vi "PTSequencer.panel.vi"() -> ()   [LabVIEW 2014, in "PTSequencer.lvlib"]
uses:
  PTSequencer.lvlib
  PTSequencer.mode.ctl
  CSlibraries/UtilityLib/UtilityLib.helpType.ctl
  CS_Core/CSSystem/CoreLib/CoreLib.string 2 byte array.vi
  CSlibraries/UtilityLib/UtilityLib.lvlib
  _common/PTUtils/PTUtils.lvlib
  CS_Core/BaseSM/BaseSM.lvlib
  CS_Core/BaseProcess/BaseProcess.lvlib
  CS_Core/CSSystem/CSSystemLib/CSSystemLib.lvlib
  CS_Core/CSSystem/CoreLib/CoreLib.lvlib
  CS_Core/CSObj/CSObj.lvlib
panel:
  out "Paused":bool
  in  "settings path":path caption="Settings file"
  out "objlist_OldVal":i32[](array[numeric])
  in  "nofLoops":u32 caption="##"
  out "Current loop":i32 caption="Loop"
  out "running":bool
  out "Current step":i32 caption="Step"
  out "State":string
  in  "Mode":T1 caption="Mode:"
  out "Busy":bool
  out "error out":errorcluster
  in  "error in (no error)":errorcluster
  in  "object ref":refnum<vi>
  out "loop counter":i32
  in  "Tab":enum32{"Sequence", "Log"}(tab)
  in  "object list":i32[](listbox)
  out "Status Log":string
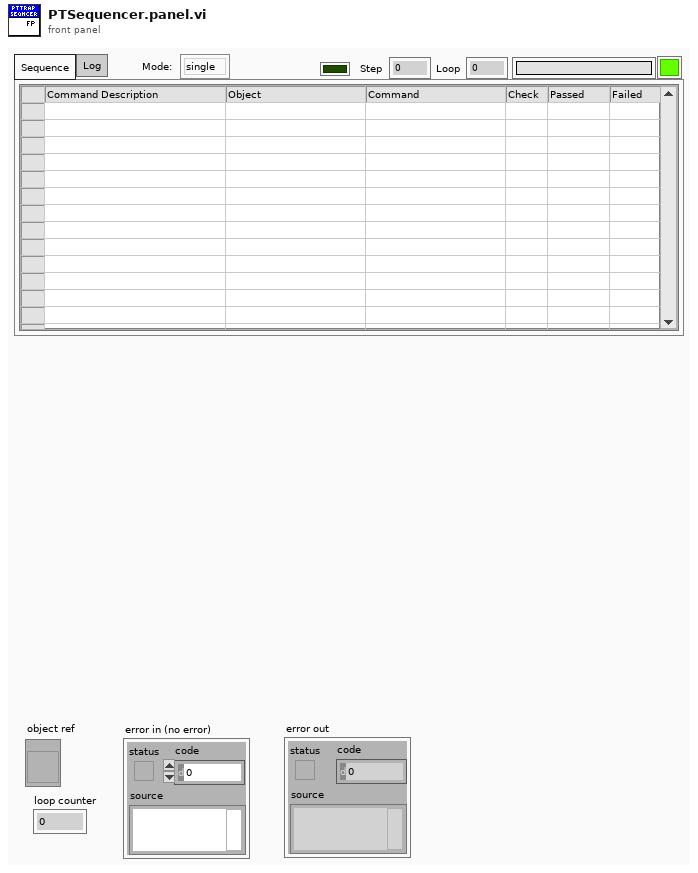
[diagram p1: front panel]
types:
  T1 = typedef "PTSequencer.lvlib/PTSequencer.mode.ctl" = enum16{"single", "loop", "for loop"}
  T2 = enum16{"open", "replace", "create", "open or create", "replace or create", "replace or create with confirmation"}
  T3 = typedef "UtilityLib.lvlib/UtilityLib.helpType.ctl" = enum16{"unknown", "menu", "description", "about", "special0", "special1", "special2"}
  T4 = typedef "PTSequencer.lvlib/PTSequencer.i attribute.ctl" = cluster{"subsequence":bool, "mode":T1, "i step":i32, "nofLoops":i32, "i loop":i32, "Running":bool, "Paused":bool, "step done":bool, "loop done":bool, "seq done":bool, "DIM IDs":cluster{"step done":i32, "loop done":i32, "seq done":i32, "i step":i32, "i loop":i32}, "use stop conditions":bool, "stop conditions":T5[], "Step List":T7[], "DIM subsriptions":string[], "stop cond indexes":i32[], "step cond indexes":cluster{"step condition IDs":cluster{"step ID":i32, "condition ID":i32}[]}[], "Delay Start Time":timestamp, "status":string, "stopping":bool}
  T5 = typedef "PTSequencer.lvlib/PTSequencer.DIM service condition.ctl" = cluster{"DIM service":string, "descr":string, "nomValue":T6, "actValue":T6, "matched":bool, "DIM Status":cluster{"no link":bool, "quality":i32, "Time Stamp":timestamp}}
  T6 = typedef "CoreDefs.rawDataType.ctl" = i8[]
  T7 = typedef "PTSequencer.lvlib/PTSequencer.step.ctl" = cluster{"description":string, "object parameters":cluster{"object":string, "selector":string, "descriptor":string, "data":T6, "subsequence":bool, "call mode":enum16{"Simple DIM", "Synchronous"}, "data in":T6}, "result action":cluster{"check":bool, "passed":enum16{"Next", "Previous", "Repeat", "Jump"}, "failed":enum16{"Next", "Previous", "Repeat", "Jump"}, "jumpID_passed":i32, "jumpID_failed":i32}, "conditions":T5[], "fulfilled ":bool, "use delay":bool, "delay time (s)":dbl, "ID":i32}
  T8 = typedef "eventvkey.ctl" = enum16{"ASCII", "Enter", "Return", "Shift", "Ctrl", "Alt", "Cmd", "Opt", "Caps", "NumLock", "Clear", "Break", "Up", "Down", "Left", "Right", "Insert", "Delete", "Home", "End", "PageUp", "PageDown", "Escape", "Help", "Pause", "ScrollLock", "F1", "F2", "F3", "F4", "F5", "F6", "F7", "F8", "F9", "F10", "F11", "F12", "F13", "F14", "F15", "F16", "F17", "F18", "F19", "F20", "F21", "F22", "F23", "F24", "Play", "VolumeUp", "VolumeDown", "Mute", "Two Byte Char"}
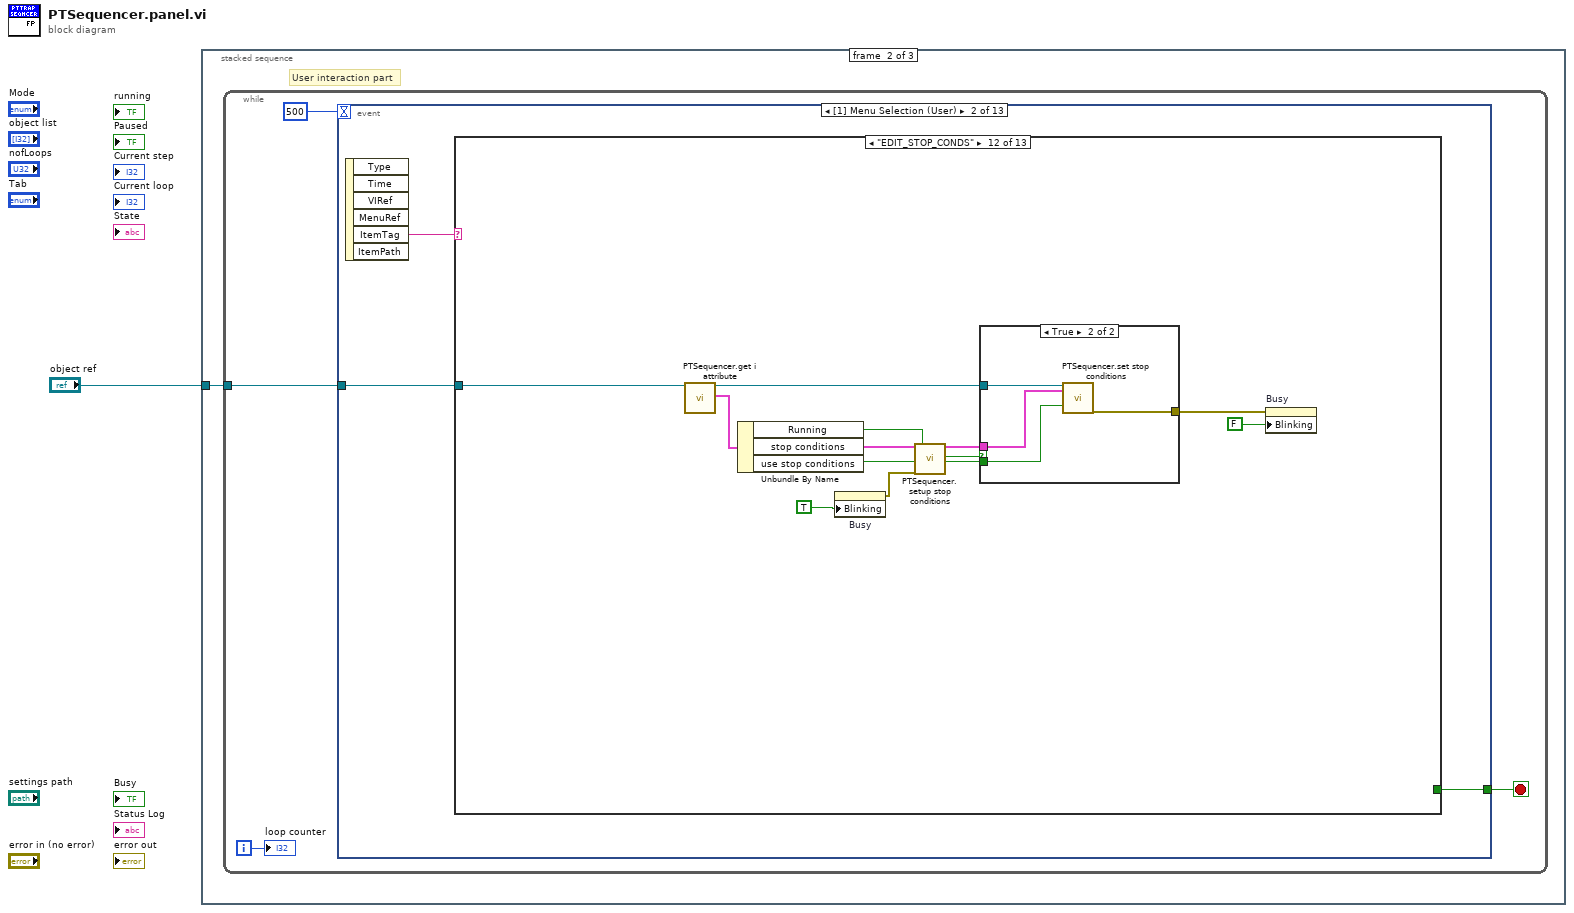
[diagram p0: block diagram]
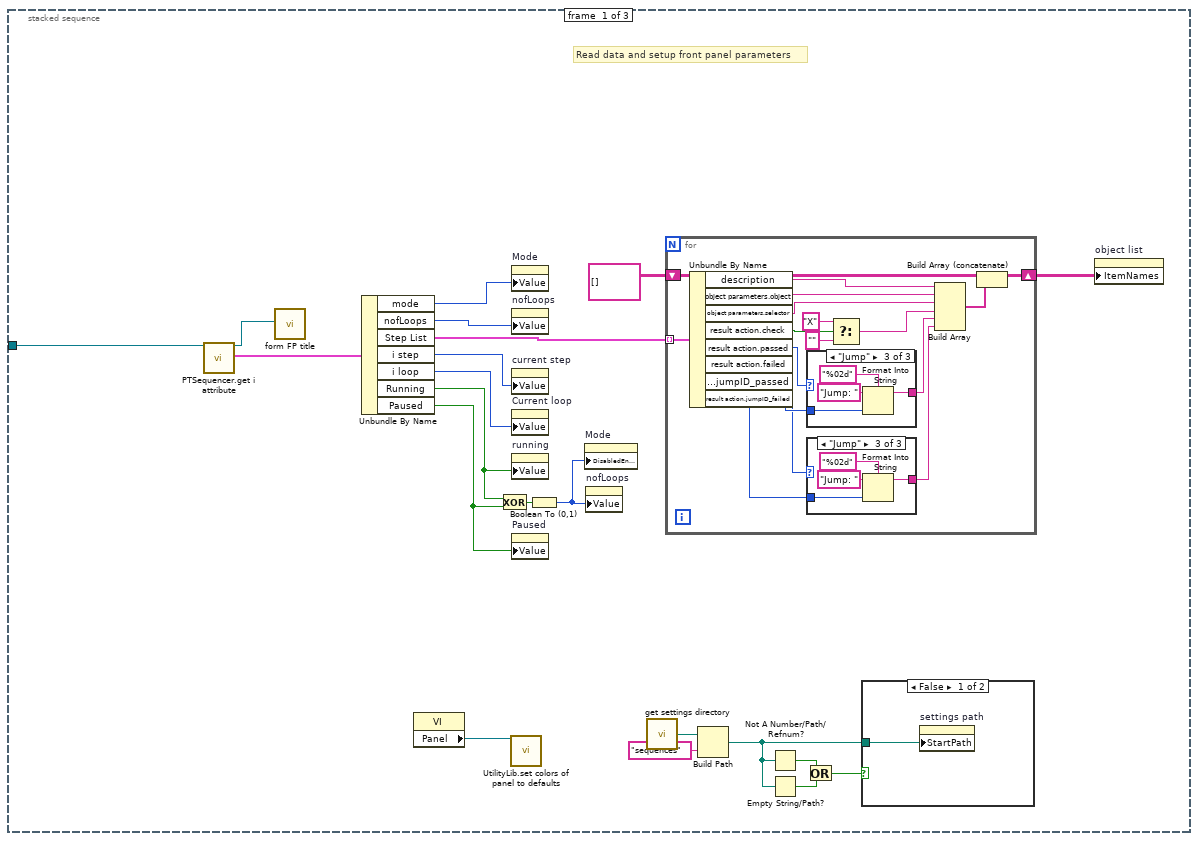
[diagram p2: hidden frame]
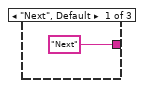
[diagram p3: hidden frame]
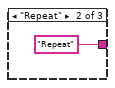
[diagram p4: hidden frame]
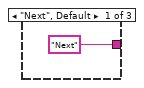
[diagram p5: hidden frame]
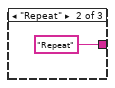
[diagram p6: hidden frame]
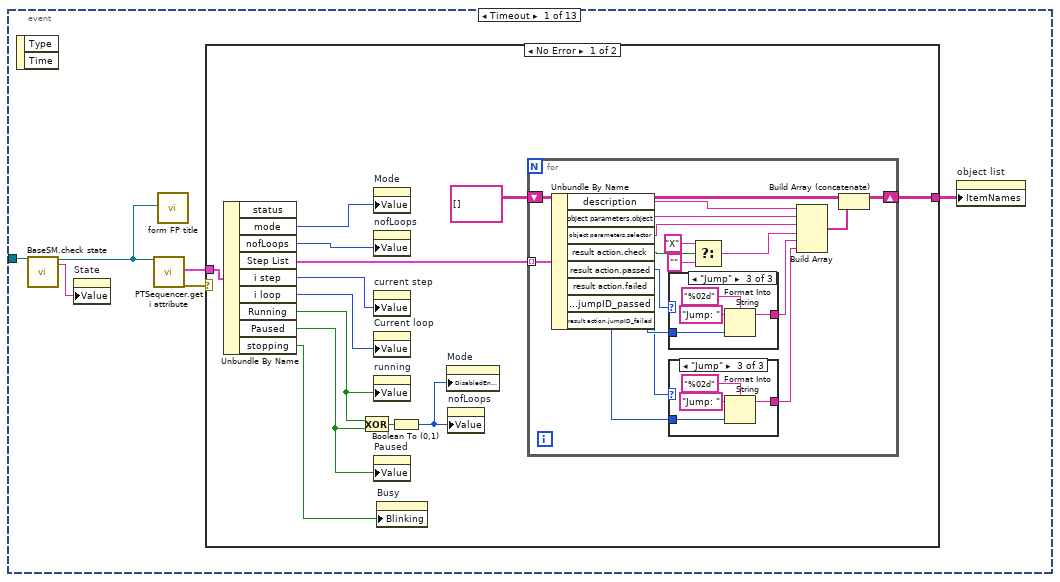
[diagram p8: hidden frame]
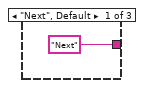
[diagram p9: hidden frame]
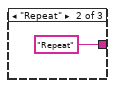
[diagram p10: hidden frame]
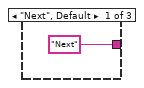
[diagram p11: hidden frame]
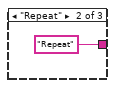
[diagram p12: hidden frame]
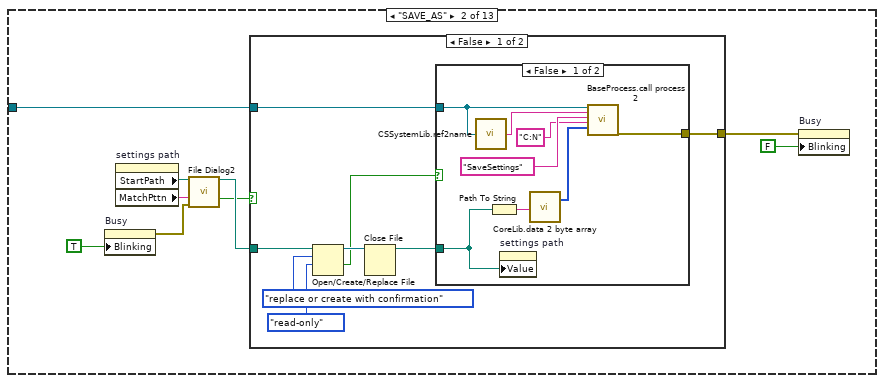
[diagram p15: hidden frame]
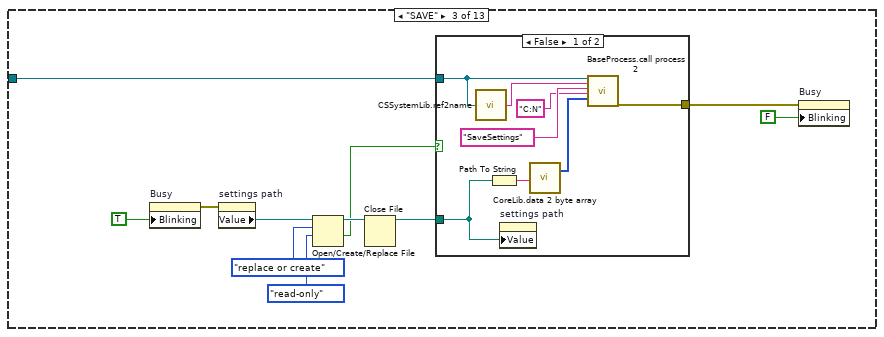
[diagram p18: hidden frame]
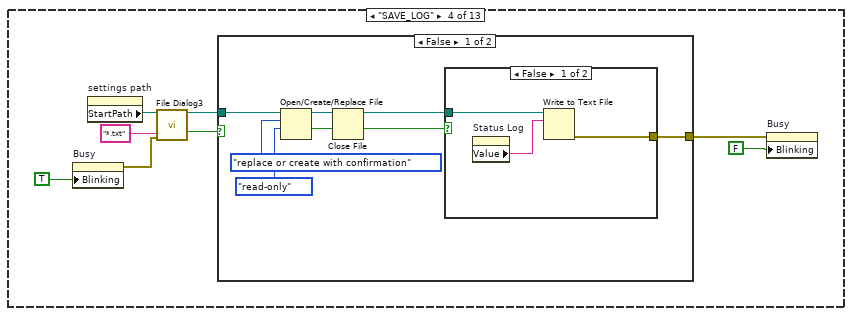
[diagram p20: hidden frame]
diagram:
  n1 = stacked-sequence {
    tunnel: "object ref" -> [w13 w53 w388]
    frame #0 {
      # "Read data and setup front panel parameters"
      n2 = call "PTSequencer.get i attribute.vi"("i ref in"=w13) -> ("i ref out"=w2:refnum<vi>, "i attribute"=w14:T4)  [unwired: 16 in, 1 out]
      n3 = call "form FP title.vi"("object ref"=w2) -> ()  [unwired: 19 in]
      n4 = Unbundle By Name(w14) -> ("mode"=w6:T1, "nofLoops"=w5:i32, "Step List"=w10:T7[], "i step"=w11:i32, "i loop"=w9:i32, "Running"=w4:bool, "Paused"=w7:bool)
      n5 = property class="VI"() -> ("Panel"=w16:refnum<vi>)  [unwired: 2 in, 2 out]
      n6 = Exclusive Or(1:w7, 2:w4) -> (0:w8:bool)
      n7 = call "UtilityLib.set colors of panel to defaults.vi"("Front Panel"=w16) -> ()  [unwired: 18 in, 1 out]
      n8 = property on="Mode" class="Enum (strict)"("Value"=w6) -> ()  [unwired: 2 in, 2 out]
      n9 = property on="nofLoops" class="DigNum (strict)"("Value"=w5) -> ()  [unwired: 2 in, 2 out]
      n10 = property on="current step" class="DigNum (strict)"("Value"=w11) -> ()  [unwired: 2 in, 2 out]
      n11 = property on="Current loop" class="DigNum (strict)"("Value"=w9) -> ()  [unwired: 2 in, 2 out]
      n12 = property on="running" class="Bool (strict)"("Value"=w4) -> ()  [unwired: 2 in, 2 out]
      n13 = property on="Paused" class="Bool (strict)"("Value"=w7) -> ()  [unwired: 2 in, 2 out]
      n14 = Boolean To (0,1)(Boolean=w8) -> (0, 1=w3:i16)
      n15 = property on="Mode" class="Enum (strict)"("DisabledEnum"=w3) -> ()  [unwired: 2 in, 2 out]
      n16 = property on="nofLoops" class="DigNum (strict)"("Value"=w3) -> ()  [unwired: 2 in, 2 out]
      n17 = call "get settings directory.vi"() -> ("settings directory"=w19:path)
      n18 = for {
        shift-right: [w38] -> w15
        shift-left: string[][] [] -> [w39]
        tunnel: w10 -> [w37] mode=indexing
        n19 = Unbundle By Name(w37) -> ("description"=w36:string, "object parameters.object"=w34:string, "object parameters.selector"=w33:string, "result action.check"=w32:bool, "result action.passed"=w27:enum16{"Next", "Previous", "Repeat", "Jump"}, "result action.failed"=w24:enum16{"Next", "Previous", "Repeat", "Jump"}, "result action.jumpID_passed"=w26:i32, "result action.jumpID_failed"=w23:i32)
        n20 = case shown="\"Jump\"" w27 {
          tunnel: ["Next" "Repeat" w50] -> w28
          tunnel: w26 -> [_ _ w49]
          frame "Next", Default {
          }
          frame "Repeat" {
          }
          frame "Jump" {
            n21 = Format Into String(format string="%02d", initial string="Jump: ", w49) -> (resulting string=w50:string)  [unwired: 1 in, 1 out]
          }
        }
        n22 = case shown="\"Jump\"" w24 {
          tunnel: ["Next" "Repeat" w44] -> w25
          tunnel: w23 -> [_ _ w43]
          frame "Next", Default {
          }
          frame "Repeat" {
          }
          frame "Jump" {
            n23 = Format Into String(format string="%02d", initial string="Jump: ", w43) -> (resulting string=w44:string)  [unwired: 1 in, 1 out]
          }
        }
        n24 = Select(t="X", s=w32, f="") -> (s? t:f=w29:string)
        n25 = Build Array(w36, w34, w33, w29, w28, w25) -> (w35:string[])
        n26 = Build Array (concatenate)(w39, w35) -> (w38:string[][])
      }
      n27 = Build Path(base path=w19, name or relative path="sequences") -> (appended path=w17:path)
      n28 = Not A Number/Path/Refnum?(number/path/refnum=w17) -> (NaN/Path/Refnum?=w22:bool)
      n29 = Empty String/Path?(string/path=w17) -> (empty?=w21:bool)
      n30 = Or(x=w22, y=w21) -> (x .or. y?=w20:bool)
      n31 = case shown="False" w20 {
        tunnel: w17 -> [w52 _]
        frame False {
          n32 = property on="settings path" class="Path"("StartPath"=w52) -> ()  [unwired: 2 in, 2 out]
        }
        frame True {
        }
      }
      n33 = property on="object list" class="MCListbox (strict)"("ItemNames"=w15) -> ()  [unwired: 2 in, 2 out]
    }
    frame #1 {
      # "User interaction part"
      n34 = while {
        tunnel: w53 -> [w54]
        i -> [w57]
        stop <- w55 stop-if-true
        n35 = event shown="[1] Menu Selection (User)" {
          selector: _ -> [_ _ _ _ _ _ _ _ _ _ _ _ _]
          dyn-events: _ -> [_ _ _ _ _ _ _ _ _ _ _ _ _]
          timeout: 500 -> [_ _ _ _ _ _ _ _ _ _ _ _ _]
          tunnel: [_ w106 _ _ _ _ _ _ _ _ _ _ _] -> w55
          tunnel: w54 -> [w63 w107 w238 _ w268 w318 w335 _ w354 w360 w369 w379 w385]
          event Timeout {
            n36 = event-data() -> ()  [unwired: 1 in, 2 out]
            n37 = call "BaseSM.check state.vi"("i ref in"=w63) -> ("i ref out"=w59:refnum<vi>, "actualState"=w60:string)  [unwired: 13 in, 4 out]
            n38 = property on="State" class="Str"("Value"=w60) -> ()  [unwired: 2 in, 2 out]
            n39 = call "PTSequencer.get i attribute.vi"("i ref in"=w59) -> ("i attribute"=w61:T4, "error out"=w58:errorcluster)  [unwired: 16 in, 1 out]
            n40 = call "form FP title.vi"("object ref"=w59) -> ()  [unwired: 19 in]
            n41 = case shown="No Error" w58 {
              tunnel: [w76 _] -> w62
              tunnel: w61 -> [w75 _]
              frame No Error {
                n42 = Unbundle By Name(w75) -> ("mode"=w68:T1, "nofLoops"=w67:i32, "Step List"=w72:T7[], "i step"=w73:i32, "i loop"=w71:i32, "Running"=w66:bool, "Paused"=w69:bool, "stopping"=w64:bool)  [unwired: 1 out]
                n43 = Exclusive Or(1:w69, 2:w66) -> (0:w70:bool)
                n44 = property on="Mode" class="Enum (strict)"("Value"=w68) -> ()  [unwired: 2 in, 2 out]
                n45 = property on="nofLoops" class="DigNum (strict)"("Value"=w67) -> ()  [unwired: 2 in, 2 out]
                n46 = property on="current step" class="DigNum (strict)"("Value"=w73) -> ()  [unwired: 2 in, 2 out]
                n47 = property on="Current loop" class="DigNum (strict)"("Value"=w71) -> ()  [unwired: 2 in, 2 out]
                n48 = property on="running" class="Bool (strict)"("Value"=w66) -> ()  [unwired: 2 in, 2 out]
                n49 = property on="Paused" class="Bool (strict)"("Value"=w69) -> ()  [unwired: 2 in, 2 out]
                n50 = property on="Busy" class="Bool (strict)"("Blinking"=w64) -> ()  [unwired: 2 in, 2 out]
                n51 = Boolean To (0,1)(Boolean=w70) -> (0, 1=w65:i16)
                n52 = property on="Mode" class="Enum (strict)"("DisabledEnum"=w65) -> ()  [unwired: 2 in, 2 out]
                n53 = property on="nofLoops" class="DigNum (strict)"("Value"=w65) -> ()  [unwired: 2 in, 2 out]
                n54 = for {
                  shift-right: [w92] -> w76
                  shift-left: string[][] [] -> [w93]
                  tunnel: w72 -> [w91] mode=indexing
                  n55 = Unbundle By Name(w91) -> ("description"=w90:string, "object parameters.object"=w88:string, "object parameters.selector"=w87:string, "result action.check"=w86:bool, "result action.passed"=w81:enum16{"Next", "Previous", "Repeat", "Jump"}, "result action.failed"=w78:enum16{"Next", "Previous", "Repeat", "Jump"}, "result action.jumpID_passed"=w80:i32, "result action.jumpID_failed"=w77:i32)
                  n56 = case shown="\"Jump\"" w81 {
                    tunnel: ["Next" "Repeat" w104] -> w82
                    tunnel: w80 -> [_ _ w103]
                    frame "Next", Default {
                    }
                    frame "Repeat" {
                    }
                    frame "Jump" {
                      n57 = Format Into String(format string="%02d", initial string="Jump: ", w103) -> (resulting string=w104:string)  [unwired: 1 in, 1 out]
                    }
                  }
                  n58 = case shown="\"Jump\"" w78 {
                    tunnel: ["Next" "Repeat" w98] -> w79
                    tunnel: w77 -> [_ _ w97]
                    frame "Next", Default {
                    }
                    frame "Repeat" {
                    }
                    frame "Jump" {
                      n59 = Format Into String(format string="%02d", initial string="Jump: ", w97) -> (resulting string=w98:string)  [unwired: 1 in, 1 out]
                    }
                  }
                  n60 = Select(t="X", s=w86, f="") -> (s? t:f=w83:string)
                  n61 = Build Array(w90, w88, w87, w83, w82, w79) -> (w89:string[])
                  n62 = Build Array (concatenate)(w93, w89) -> (w92:string[][])
                }
              }
              frame Error {
              }
            }
            n63 = property on="object list" class="MCListbox (strict)"("ItemNames"=w62) -> ()  [unwired: 2 in, 2 out]
          }
          event Menu Selection (User) {
            n64 = event-data() -> ("ItemTag"=w108:string)  [unwired: 1 in, 5 out]
            n65 = case shown="\"EDIT_STOP_CONDS\"" w108 {
              tunnel: w107 -> [_ w113 w144 _ w182 _ w193 w195 w198 w201 w206 w223 _]
              tunnel: [_ _ _ _ _ TRUE _ _ _ _ _ _ _] -> w106
              frame "", Default {
              }
              frame "SAVE_AS" {
                n66 = property on="Busy" class="Bool (strict)"("Blinking"=TRUE) -> (error out=w109:errorcluster)  [unwired: 2 in, 1 out]
                n67 = property on="settings path" class="Path"() -> ("StartPath"=w117:path, "MatchPttn"=w116:string)  [unwired: 2 in, 2 out]
                n68 = call "File Dialog2"("start path"=w117, "error in"=w109, "pattern (all files)"=w116) -> ("selected path"=w115:path, "cancelled"=w114:bool)  [unwired: 9 in, 2 out]
                n69 = case shown="False" w114 {
                  tunnel: w115 -> [w124 _]
                  tunnel: w113 -> [w125 _]
                  tunnel: [w118 _] -> w111
                  frame False {
                    n70 = Open/Create/Replace File(file path (use dialog)=w124, operation (0:open)=T2."replace or create with confirmation", access (0:read/write)=enum16{"read/write", "read-only", "write-only"}."read-only") -> (refnum out=w123:refnum<file>, cancelled=w121:bool)  [unwired: 3 in, 1 out]
                    n71 = Close File(refnum=w123) -> (path=w122:path)  [unwired: 1 in, 1 out]
                    n72 = case shown="False" w121 {
                      tunnel: w122 -> [w127 _]
                      tunnel: w125 -> [w129 _]
                      tunnel: [w126 _] -> w118
                      frame False {
                        n73 = call "CSSystemLib.ref2name.vi"("obj refnum"=w129) -> ("name"=w128:string)
                        n74 = Path To String(path=w127) -> (string=w130:string)
                        n75 = property on="settings path" class="Path"("Value"=w127) -> ()  [unwired: 2 in, 2 out]
                        n76 = call-poly "CoreLib.data 2 byte array.vi"("string"=w130) -> ("byteArray out"=w131:T6)  [unwired: 18 in]
                        n77 = call "BaseProcess.call process 2.vi"("i ref in"=w129, "Object"=w128, "Selector"="SaveSettings", "Data Descriptor"="C:N", "Data"=w131) -> ("error out"=w126:errorcluster)  [unwired: 13 in, 1 out]
                      }
                      frame True {
                      }
                    }
                  }
                  frame True {
                  }
                }
                n78 = property on="Busy" class="Bool (strict)"(error in=w111, "Blinking"=FALSE) -> ()  [unwired: 1 in, 2 out]
              }
              frame "SAVE" {
                n79 = property on="Busy" class="Bool (strict)"("Blinking"=TRUE) -> (error out=w139:errorcluster)  [unwired: 2 in, 1 out]
                n80 = property on="settings path" class="Path"(error in=w139) -> ("Value"=w140:path)  [unwired: 1 in, 2 out]
                n81 = Open/Create/Replace File(file path (use dialog)=w140, operation (0:open)=T2."replace or create", access (0:read/write)=enum16{"read/write", "read-only", "write-only"}."read-only") -> (refnum out=w138:refnum<file>, cancelled=w136:bool)  [unwired: 3 in, 1 out]
                n82 = Close File(refnum=w138) -> (path=w137:path)  [unwired: 1 in, 1 out]
                n83 = case shown="False" w136 {
                  tunnel: w137 -> [w146 _]
                  tunnel: w144 -> [w148 _]
                  tunnel: [w145 _] -> w142
                  frame False {
                    n84 = call "CSSystemLib.ref2name.vi"("obj refnum"=w148) -> ("name"=w147:string)
                    n85 = Path To String(path=w146) -> (string=w149:string)
                    n86 = property on="settings path" class="Path"("Value"=w146) -> ()  [unwired: 2 in, 2 out]
                    n87 = call-poly "CoreLib.data 2 byte array.vi"("string"=w149) -> ("byteArray out"=w150:T6)  [unwired: 18 in]
                    n88 = call "BaseProcess.call process 2.vi"("i ref in"=w148, "Object"=w147, "Selector"="SaveSettings", "Data Descriptor"="C:N", "Data"=w150) -> ("error out"=w145:errorcluster)  [unwired: 13 in, 1 out]
                  }
                  frame True {
                  }
                }
                n89 = property on="Busy" class="Bool (strict)"(error in=w142, "Blinking"=FALSE) -> ()  [unwired: 1 in, 2 out]
              }
              frame "SAVE_LOG" {
                n90 = property on="Busy" class="Bool (strict)"("Blinking"=TRUE) -> (error out=w154:errorcluster)  [unwired: 2 in, 1 out]
                n91 = property on="settings path" class="Path"() -> ("StartPath"=w160:path)  [unwired: 2 in, 2 out]
                n92 = call "File Dialog3"("start path"=w160, "error in"=w154, "pattern (all files)"="*.txt" ("default name")) -> ("selected path"=w159:path, "cancelled"=w158:bool)  [unwired: 9 in, 2 out]
                n93 = case shown="False" w158 {
                  tunnel: w159 -> [w167 _]
                  tunnel: [w161 _] -> w156
                  frame False {
                    n94 = Open/Create/Replace File(file path (use dialog)=w167, operation (0:open)=T2."replace or create with confirmation", access (0:read/write)=enum16{"read/write", "read-only", "write-only"}."read-only") -> (refnum out=w166:refnum<file>, cancelled=w164:bool)  [unwired: 3 in, 1 out]
                    n95 = Close File(refnum=w166) -> (path=w165:path)  [unwired: 1 in, 1 out]
                    n96 = case shown="False" w164 {
                      tunnel: w165 -> [w168 _]
                      tunnel: [w169 _] -> w161
                      frame False {
                        n97 = property on="Status Log" class="Str"() -> ("Value"=w170:string)  [unwired: 2 in, 2 out]
                        n98 = Write to Text File(file (use dialog)=w168, text=w170) -> (error out=w169:errorcluster)  [unwired: 2 in, 2 out]
                      }
                      frame True {
                      }
                    }
                  }
                  frame True {
                  }
                }
                n99 = property on="Busy" class="Bool (strict)"(error in=w156, "Blinking"=FALSE) -> ()  [unwired: 1 in, 2 out]
              }
              frame "LOAD" {
                n100 = property on="settings path" class="Path"() -> ("StartPath"=w181:path, "MatchPttn"=w180:string)  [unwired: 2 in, 2 out]
                n101 = property on="Busy" class="Bool (strict)"("Blinking"=TRUE) -> (error out=w171:errorcluster)  [unwired: 2 in, 1 out]
                n102 = call "File Dialog"("start path"=w181, "error in"=w171, "pattern (all files)"=w180) -> ("selected path"=w179:path, "exists"=w175:bool, "cancelled"=w177:bool)  [unwired: 9 in, 1 out]
                n103 = Not(x=w175) -> (.not. x?=w178:bool)
                n104 = Or(x=w178, y=w177) -> (x .or. y?=w176:bool)
                n105 = case shown="False" w176 {
                  tunnel: w182 -> [w187 _]
                  tunnel: w179 -> [w185 _]
                  tunnel: [w183 _] -> w172
                  frame False {
                    n106 = call "CSSystemLib.ref2name.vi"("obj refnum"=w187) -> ("name"=w188:string)
                    n107 = Path To String(path=w185) -> (string=w186:string)
                    n108 = property on="settings path" class="Path"("Value"=w185) -> ()  [unwired: 2 in, 2 out]
                    n109 = call-poly "CoreLib.data 2 byte array.vi"("string"=w186) -> ("byteArray out"=w189:T6)  [unwired: 18 in]
                    n110 = call "BaseProcess.call process 1.vi"("i ref in"=w187, "Object"=w188, "Selector"="LoadSettings", "CallType"=enum16{"simple", "synchronous", "asynchronous"}."synchronous", "Data"=w189, "Data Descriptor"="C:N") -> ("error out"=w183:errorcluster)  [unwired: 11 in, 2 out]
                  }
                  frame True {
                  }
                }
                n111 = property on="Busy" class="Bool (strict)"(error in=w172, "Blinking"=FALSE) -> ()  [unwired: 1 in, 2 out]
              }
              frame "QUIT" {
              }
              frame "Hide" {
                n112 = call "CSObj.open front panel.vi"("i ref in"=w193, "frontPanelOpen"=FALSE ("front panel open")) -> ()  [unwired: 16 in, 2 out]
              }
              frame "START" {
                n113 = call "CSSystemLib.ref2name.vi"("obj refnum"=w195) -> ("name"=w197:string)
                n114 = call "BaseProcess.call process 2.vi"("i ref in"=w195, "Object"=w197, "Selector"="Start") -> ()  [unwired: 15 in, 2 out]
              }
              frame "STOP" {
                n115 = call "CSSystemLib.ref2name.vi"("obj refnum"=w198) -> ("name"=w200:string)
                n116 = call "BaseProcess.call process 2.vi"("i ref in"=w198, "Object"=w200, "Selector"="Stop") -> ()  [unwired: 15 in, 2 out]
              }
              frame "ABORT" {
                n117 = call "CSSystemLib.ref2name.vi"("obj refnum"=w201) -> ("name"=w203:string)
                n118 = call "BaseProcess.call process 2.vi"("i ref in"=w201, "Object"=w203, "Selector"="Abort") -> ()  [unwired: 15 in, 2 out]
              }
              frame "PAUSE" {
                n119 = property on="Paused" class="Bool (strict)"() -> ("Value"=w205:bool)  [unwired: 2 in, 2 out]
                n120 = Not(x=w205) -> (.not. x?=w204:bool)
                n121 = case shown="True" w204 {
                  tunnel: w206 -> [w209 w212]
                  frame True {
                    n122 = call "CSSystemLib.ref2name.vi"("obj refnum"=w209) -> ("name"=w208:string)
                    n123 = call "BaseProcess.call process 2.vi"("i ref in"=w209, "Object"=w208, "Selector"="Pause") -> ()  [unwired: 15 in, 2 out]
                  }
                  frame False {
                    n124 = call "CSSystemLib.ref2name.vi"("obj refnum"=w212) -> ("name"=w211:string)
                    n125 = call "BaseProcess.call process 2.vi"("i ref in"=w212, "Object"=w211, "Selector"="Start") -> ()  [unwired: 15 in, 2 out]
                  }
                }
              }
              frame "EDIT_STOP_CONDS" {
                n126 = call "PTSequencer.get i attribute.vi"("i ref in"=w223) -> ("i ref out"=w224:refnum<vi>, "i attribute"=w225:T4)  [unwired: 16 in, 1 out]
                n127 = Unbundle By Name(w225) -> ("Running"=w213:bool, "stop conditions"=w220:T5[], "use stop conditions"=w219:bool)
                n128 = property on="Busy" class="Bool (strict)"("Blinking"=TRUE) -> (error out=w214:errorcluster)  [unwired: 2 in, 1 out]
                n129 = call "PTSequencer.setup stop conditions.vi"("stop conditions in"=w220, "Use stop conditions in"=w219, "error in (no error)"=w214, "read only"=w213) -> ("stop conditions out"=w217:T5[], "changed"=w216:bool, "Use stop conditions out"=w218:bool)  [unwired: 12 in, 1 out]
                n130 = case shown="True" w216 {
                  tunnel: w218 -> [_ w228]
                  tunnel: w217 -> [_ w229]
                  tunnel: w224 -> [_ w227]
                  tunnel: [_ w226] -> w221
                  frame False {
                  }
                  frame True {
                    n131 = call "PTSequencer.set stop conditions.vi"("i ref in"=w227, "stop conditions"=w229, "use stop conditions"=w228) -> ("error out"=w226:errorcluster)  [unwired: 14 in, 2 out]
                  }
                }
                n132 = property on="Busy" class="Bool (strict)"(error in=w221, "Blinking"=FALSE) -> ()  [unwired: 1 in, 2 out]
              }
              frame "helpDescription" {
                n133 = call "UtilityLib.show help.vi"("helpType"=UtilityLib.helpType."description") -> ()
              }
            }
          }
          event Menu Activation? {
            n134 = event-data() -> ("MenuRef"=w244:refnum<k9>)  [unwired: 1 in, 3 out]
            n135 = call "PTSequencer.get i attribute.vi"("i ref in"=w238) -> ("i attribute"=w237:T4)  [unwired: 16 in, 2 out]
            n136 = Unbundle By Name(w237) -> ("Step List"=w236:T7[])
            n137 = Array Size(array=w236) -> (size(s)=w235:i32)
            n138 = Greater Than 0?(x=w235) -> (x > 0?=w234:bool)
            n139 = property on="running" class="Bool (strict)"() -> ("Value"=w253:bool)  [unwired: 2 in, 2 out]
            n140 = property on="settings path" class="Path"() -> ("Value"=w240:path)  [unwired: 2 in, 2 out]
            n141 = Empty String/Path?(string/path=w240) -> (empty?=w242:bool)
            n142 = Not A Number/Path/Refnum?(number/path/refnum=w240) -> (NaN/Path/Refnum?=w241:bool)
            n143 = Not(x=w253) -> (.not. x?=w239:bool)
            n144 = Not Or(1:w241, 2:w242) -> (0:w233:bool)
            n145 = And(x=w234, y=w239) -> (x .and. y?=w232:bool)
            n146 = And(x=w233, y=w232) -> (x .and. y?=w231:bool)
            n147 = Set Menu Item Info(7:"SAVE", 9:w231, 11:w244) -> (3:w243:refnum<k9>)  [unwired: 4 in, 1 out]
            n148 = Set Menu Item Info(7:"SAVE_AS", 9:w232, 11:w243) -> (3:w256:refnum<k9>)  [unwired: 4 in, 1 out]
            n149 = property on="Status Log" class="Str"() -> ("Value"=w250:string)  [unwired: 2 in, 2 out]
            n150 = Set Menu Item Info(7:"LOAD", 9:w239, 11:w256) -> (3:w252:refnum<k9>)  [unwired: 4 in, 1 out]
            n151 = call <vilib>:"Trim Whitespace.vi"("string"=w250) -> ("trimmed string"=w251:string)  [unwired: 1 in]
            n152 = property on="Paused" class="Bool (strict)"() -> ("Value"=w254:bool)  [unwired: 2 in, 2 out]
            n153 = Empty String/Path?(string/path=w251) -> (empty?=w247:bool)
            n154 = Set Menu Item Info(6:w254, 7:"PAUSE", 9:w253, 11:w252) -> (3:w248:refnum<k9>)  [unwired: 3 in, 1 out]
            n155 = Not(x=w247) -> (.not. x?=w246:bool)
            n156 = Set Menu Item Info(7:"SAVE_LOG", 9:w246, 11:w248) -> ()  [unwired: 4 in, 2 out]
            n157 = event-data() -> ()  [unwired: 2 in, 1 out]
          }
          event "object list": Shortcut Menu Activation? {
            n158 = event-data() -> ("MenuRef"=w259:refnum<k9>)  [unwired: 1 in]
            n159 = property on="object list" class="MCListbox (strict)"() -> ("Value"=w261:i32[])  [unwired: 2 in, 2 out]
            n160 = Array Size(array=w261) -> (size(s)=w260:i32)
            n161 = case shown="0, Default" w260 {
              tunnel: w259 -> [w263 w266]
              frame 0, Default {
                n162 = Set Menu Item Info(7:"CMD_EDIT", 9:FALSE, 11:w263) -> ()  [unwired: 4 in, 2 out]
              }
              frame 1 {
                n163 = Set Menu Item Info(7:"CMD_EDIT", 9:TRUE, 11:w266) -> ()  [unwired: 4 in, 2 out]
              }
            }
            n164 = event-data() -> ()  [unwired: 2 in, 1 out]
          }
          event "object list": Shortcut Menu Selection (User) {
            n165 = event-data() -> ("ItemTag"=w269:string)  [unwired: 1 in]
            n166 = case shown="\"CMD_EDIT\", Default" w269 {
              tunnel: w268 -> [w279 w288 w307 w314]
              frame "CMD_ADD" {
                n167 = call "PTSequencer.get i attribute.vi"("i ref in"=w279) -> ("i ref out"=w276:refnum<vi>, "i attribute"=w277:T4)  [unwired: 16 in, 1 out]
                n168 = property on="Busy" class="Bool (strict)"("Blinking"=TRUE) -> (error out=w272:errorcluster)  [unwired: 2 in, 1 out]
                n169 = Unbundle By Name(w277) -> ("Step List"=w278:T7[])
                n170 = call "PTSequencer.dialog edit step.vi"("Step List In"=w278, "new"=TRUE, "error in (no error)"=w272) -> ("Step Out"=w275:T7, "changed"=w274:bool)  [unwired: 13 in, 2 out]
                n171 = case shown="True" w274 {
                  tunnel: w276 -> [_ w283]
                  tunnel: w275 -> [_ w282]
                  tunnel: [_ w281] -> w270
                  frame False {
                  }
                  frame True {
                    n172 = call "PTSequencer.add step.vi"("i ref in"=w283, "Step"=w282) -> ("error out"=w281:errorcluster)  [unwired: 15 in, 2 out]
                  }
                }
                n173 = property on="Busy" class="Bool (strict)"(error in=w270, "Blinking"=FALSE) -> ()  [unwired: 1 in, 2 out]
              }
              frame "CMD_EDIT", Default {
                n174 = property on="object list" class="MCListbox (strict)"() -> ("Value"=w286:i32[])  [unwired: 2 in, 2 out]
                n175 = Array Size(array=w286) -> (size(s)=w287:i32)
                n176 = case shown="1" w287 {
                  tunnel: w288 -> [_ w299]
                  tunnel: w286 -> [_ w293]
                  tunnel: [_ w289] -> w284
                  frame 0, Default {
                  }
                  frame 1 {
                    n177 = Index Array(array=w293) -> (element=w292:i32)  [unwired: 1 in]
                    n178 = call "PTSequencer.get i attribute.vi"("i ref in"=w299) -> ("i ref out"=w296:refnum<vi>, "i attribute"=w297:T4)  [unwired: 16 in, 1 out]
                    n179 = Unbundle By Name(w297) -> ("Step List"=w298:T7[])
                    n180 = property on="Busy" class="Bool (strict)"("Blinking"=TRUE) -> (error out=w290:errorcluster)  [unwired: 2 in, 1 out]
                    n181 = call "PTSequencer.dialog edit step.vi"("Step List In"=w298, "i step"=w292, "new"=FALSE, "error in (no error)"=w290) -> ("Step Out"=w295:T7, "changed"=w294:bool)  [unwired: 12 in, 2 out]
                    n182 = case shown="True" w294 {
                      tunnel: w296 -> [_ w304]
                      tunnel: w295 -> [_ w303]
                      tunnel: w292 -> [_ w302]
                      tunnel: [_ w301] -> w289
                      frame False {
                      }
                      frame True {
                        n183 = call "PTSequencer.edit step.vi"("i ref in"=w304, "Step"=w303, "index"=w302) -> ("error out"=w301:errorcluster)  [unwired: 14 in, 2 out]
                      }
                    }
                  }
                }
                n184 = property on="Busy" class="Bool (strict)"(error in=w284, "Blinking"=FALSE) -> ()  [unwired: 1 in, 2 out]
              }
              frame "CMD_DELETE" {
                n185 = property on="object list" class="MCListbox (strict)"() -> ("Value"=w306:i32[])  [unwired: 2 in, 2 out]
                n186 = Reverse 1D Array(array=w306) -> (reversed array=w305:i32[])
                n187 = for {
                  tunnel: w305 -> [w309] mode=indexing
                  tunnel: w307 -> [w308]
                  n188 = call "PTSequencer.remove step.vi"("i ref in"=w308, "index"=w309) -> ()  [unwired: 15 in, 3 out]
                }
              }
              frame "CLEAR_LIST" {
                n189 = Two Button Dialog(message="Clear object list?", 1:"No", 2:"Yes") -> (T button?=w310:bool)
                n190 = case shown="True" w310 {
                  tunnel: w314 -> [_ w315]
                  frame False {
                  }
                  frame True {
                    n191 = call "PTSequencer.clear list.vi"("i ref in"=w315) -> ()  [unwired: 16 in, 3 out]
                  }
                }
              }
            }
          }
          event "object list": Key Down? {
            n192 = event-data() -> ("VKey"=w317:T8)  [unwired: 1 in]
            n193 = case shown="\"Delete\"" w317 {
              tunnel: w318 -> [w321 _]
              tunnel: [_ TRUE] -> w316
              frame "Delete" {
                n194 = call "PTSequencer.get i attribute.vi"("i ref in"=w321) -> ("i ref out"=w320:refnum<vi>, "i attribute"=w324:T4)  [unwired: 16 in, 1 out]
                n195 = Unbundle By Name(w324) -> ("Running"=w323:bool, "Paused"=w322:bool)
                n196 = Exclusive Or(1:w322, 2:w323) -> (0:w319:bool)
                n197 = case shown="False" w319 {
                  tunnel: w320 -> [w325 _]
                  frame False {
                    n198 = property on="object list" class="MCListbox (strict)"() -> ("Value"=w327:i32[])  [unwired: 2 in, 2 out]
                    n199 = Reverse 1D Array(array=w327) -> (reversed array=w326:i32[])
                    n200 = for {
                      tunnel: w326 -> [w329] mode=indexing
                      tunnel: w325 -> [w328]
                      n201 = call "PTSequencer.remove step.vi"("i ref in"=w328, "index"=w329) -> ()  [unwired: 15 in, 3 out]
                    }
                  }
                  frame True {
                  }
                }
              }
              frame Default {
              }
            }
            n202 = event-data("Discard?"=w316) -> ()  [unwired: 1 in, 1 out]
          }
          event "object list": Double Click {
            n203 = event-data() -> ()  [unwired: 1 in, 8 out]
            n204 = property on="object list" class="MCListbox (strict)"() -> ("Value"=w333:i32[])  [unwired: 2 in, 2 out]
            n205 = Array Size(array=w333) -> (size(s)=w334:i32)
            n206 = case shown="1" w334 {
              tunnel: w335 -> [_ w347]
              tunnel: w333 -> [_ w342]
              tunnel: [_ w338] -> w331
              frame 0, Default {
              }
              frame 1 {
                n207 = Index Array(array=w342) -> (element=w341:i32)  [unwired: 1 in]
                n208 = call "PTSequencer.get i attribute.vi"("i ref in"=w347) -> ("i ref out"=w344:refnum<vi>, "i attribute"=w345:T4)  [unwired: 16 in, 1 out]
                n209 = Unbundle By Name(w345) -> ("Running"=w337:bool, "Step List"=w346:T7[])
                n210 = property on="Busy" class="Bool (strict)"("Blinking"=TRUE) -> (error out=w339:errorcluster)  [unwired: 2 in, 1 out]
                n211 = call "PTSequencer.dialog edit step.vi"("Step List In"=w346, "i step"=w341, "new"=FALSE, "error in (no error)"=w339, "read only"=w337) -> ("Step Out"=w343:T7, "changed"=w336:bool)  [unwired: 11 in, 2 out]
                n212 = case shown="True" w336 {
                  tunnel: w344 -> [_ w352]
                  tunnel: w343 -> [_ w351]
                  tunnel: w341 -> [_ w350]
                  tunnel: [_ w349] -> w338
                  frame False {
                  }
                  frame True {
                    n213 = call "PTSequencer.edit step.vi"("i ref in"=w352, "Step"=w351, "index"=w350) -> ("error out"=w349:errorcluster)  [unwired: 14 in, 2 out]
                  }
                }
              }
            }
            n214 = property on="Busy" class="Bool (strict)"(error in=w331, "Blinking"=FALSE) -> ()  [unwired: 1 in, 2 out]
          }
          event "object list": Value Change {
            n215 = event-data() -> ("OldVal"=→"objlist_OldVal":i32[])  [unwired: 1 in]
          }
          event "object list": Drag Ended {
            n216 = event-data() -> ("Result"=w355:enum16{"Drop Cancel", "Drop Move", "Drop Copy"})  [unwired: 1 in]
            n217 = case shown="\"Drop Move\"" w355 {
              tunnel: w354 -> [_ w358]
              frame "Drop Cancel", Default {
              }
              frame "Drop Move" {
                n218 = property on="objlist_OldVal" class="Arr (strict)"() -> ("Value"=w357:i32[])  [unwired: 2 in, 2 out]
                n219 = property on="object list" class="MCListbox (strict)"() -> ("Value"=w356:i32[])  [unwired: 2 in, 2 out]
                n220 = call "PTSequencer.swap steps.vi"("i ref in"=w358, "old indexes"=w357, "new indexes"=w356) -> ()  [unwired: 14 in, 3 out]
              }
            }
          }
          event "object list": Drag Starting? {
            n221 = event-data() -> ()  [unwired: 1 in, 5 out]
            n222 = call "PTSequencer.get i attribute.vi"("i ref in"=w360) -> ("i attribute"=w363:T4)  [unwired: 16 in, 2 out]
            n223 = Unbundle By Name(w363) -> ("Running"=w362:bool, "Paused"=w361:bool)
            n224 = Exclusive Or(1:w361, 2:w362) -> (0:w359:bool)
            n225 = event-data("Discard?"=w359) -> ()  [unwired: 1 in, 1 out]
          }
          event Value Change {
            n226 = event-data() -> ("NewVal"=w365:T1)  [unwired: 1 in]
            n227 = case shown="\"loop\"" w365 {
              tunnel: [_ _ TRUE] -> w364
              frame "single", Default {
              }
              frame "loop" {
              }
              frame "for loop" {
              }
            }
            n228 = property on="nofLoops" class="DigNum (strict)"("Visible"=w364) -> ()  [unwired: 2 in, 2 out]
            n229 = call "PTSequencer.get data to modify.vi"("i ref in"=w369) -> ("i ref out"=w366:refnum<vi>, "i attribute"=w367:T4, "timed out"=w368:bool)  [unwired: 15 in, 1 out]
            n230 = case shown="True" w368 {
              tunnel: w367 -> [w371 _]
              tunnel: w366 -> [w374 _]
              tunnel: w365 -> [w372 _]
              frame False {
                n231 = Bundle By Name(cluster=w371, "mode"=w372) -> (w373:T4)
                n232 = call "PTSequencer.set modified data.vi"("i ref in"=w374, "CLASS.i attribute"=w373) -> ()  [unwired: 16 in, 2 out]
              }
              frame True {
              }
            }
          }
          event "nofLoops": Value Change {
            n233 = event-data() -> ("NewVal"=w375:u32)  [unwired: 1 in]
            n234 = call "PTSequencer.get data to modify.vi"("i ref in"=w379) -> ("i ref out"=w376:refnum<vi>, "i attribute"=w377:T4, "timed out"=w378:bool)  [unwired: 15 in, 1 out]
            n235 = case shown="False" w378 {
              tunnel: w377 -> [w382 _]
              tunnel: w376 -> [w384 _]
              tunnel: w375 -> [w381 _]
              frame False {
                n236 = To Long Integer(number=w381) -> (32bit integer=w380:i32)
                n237 = Bundle By Name(cluster=w382, "nofLoops"=w380) -> (w383:T4)
                n238 = call "PTSequencer.set modified data.vi"("i ref in"=w384, "CLASS.i attribute"=w383) -> ()  [unwired: 16 in, 2 out]
              }
              frame True {
              }
            }
          }
          event Panel Close? {
            n239 = event-data() -> ()  [unwired: 1 in, 3 out]
            n240 = call "CSObj.open front panel.vi"("i ref in"=w385, "frontPanelOpen"=FALSE ("front panel open")) -> ()  [unwired: 16 in, 2 out]
            n241 = event-data() -> ()  [unwired: 2 in, 1 out]
          }
        }
        "loop counter" <- w57
      }
    }
    frame #2 {
      # "Close panel - run GOG destructor"
      n242 = call "destroy this.vi"("i ref in"=w388, "close FP first"=TRUE) -> ()  [unwired: 17 in, 1 out]
    }
  }
